vi "Compound Variant to Array of Variants.vi"(8 "error in (no error)":errorcluster, 11 "Array/Cluster Variant":variant) -> (0 "error out":errorcluster, 3 "[Variant]":variant[](array[variant]))   [LabVIEW 2018, in "Potentiostat Galvanostat.lvclass"]
uses:
  Potentiostat Galvanostat.lvclass
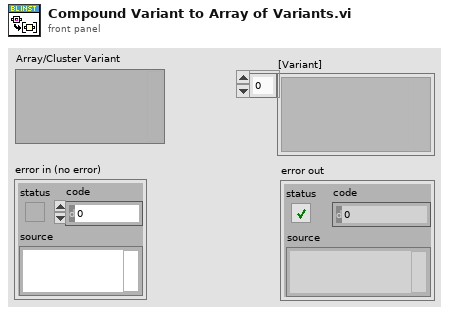
[diagram p1: front panel]
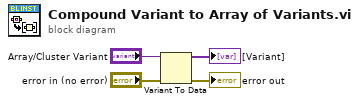
[diagram p0: block diagram]
diagram:
  n1 = Variant To Data(error in="error in (no error)", Variant="Array/Cluster Variant") -> (data=→"[Variant]":variant[], error out=→"error out":errorcluster)  [unwired: 1 in]
